vi "Reset.vi"(8 "error in (no error)":errorcluster, 11 "Session Handle":refnum<k15>) -> (0 "error out":errorcluster, 3 "Session Handle Out":refnum<k15>)   [LabVIEW 2026, in "PXI4072.lvlib"]
uses:
  PXI4072.lvlib
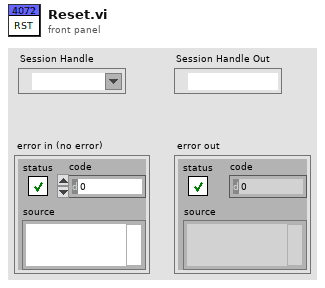
[diagram p1: front panel]
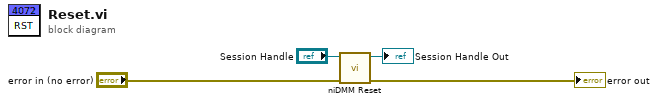
[diagram p0: block diagram]
diagram:
  n1 = call <instrlib>:"niDMM Reset.vi"("error in (no error)"="error in (no error)", "instrument handle"="Session Handle") -> ("error out"=→"error out":errorcluster, "instrument handle out"=→"Session Handle Out":refnum<k15>)  [unwired: 8 in]
